vi "Write file.vi"() -> ()   [LabVIEW 2019]
panel:
  out "text":string
  in  "stop":bool
  in  "Enable 3":bool=TRUE caption="Enable"
  out "AZ1 Actual Current (A)":dbl format="%.2f"
  out "AZ2 EN ST":bool=TRUE
  out "AZ Axis POS (Arecsec)":dbl
  out "AZ1 EN ST":bool=TRUE
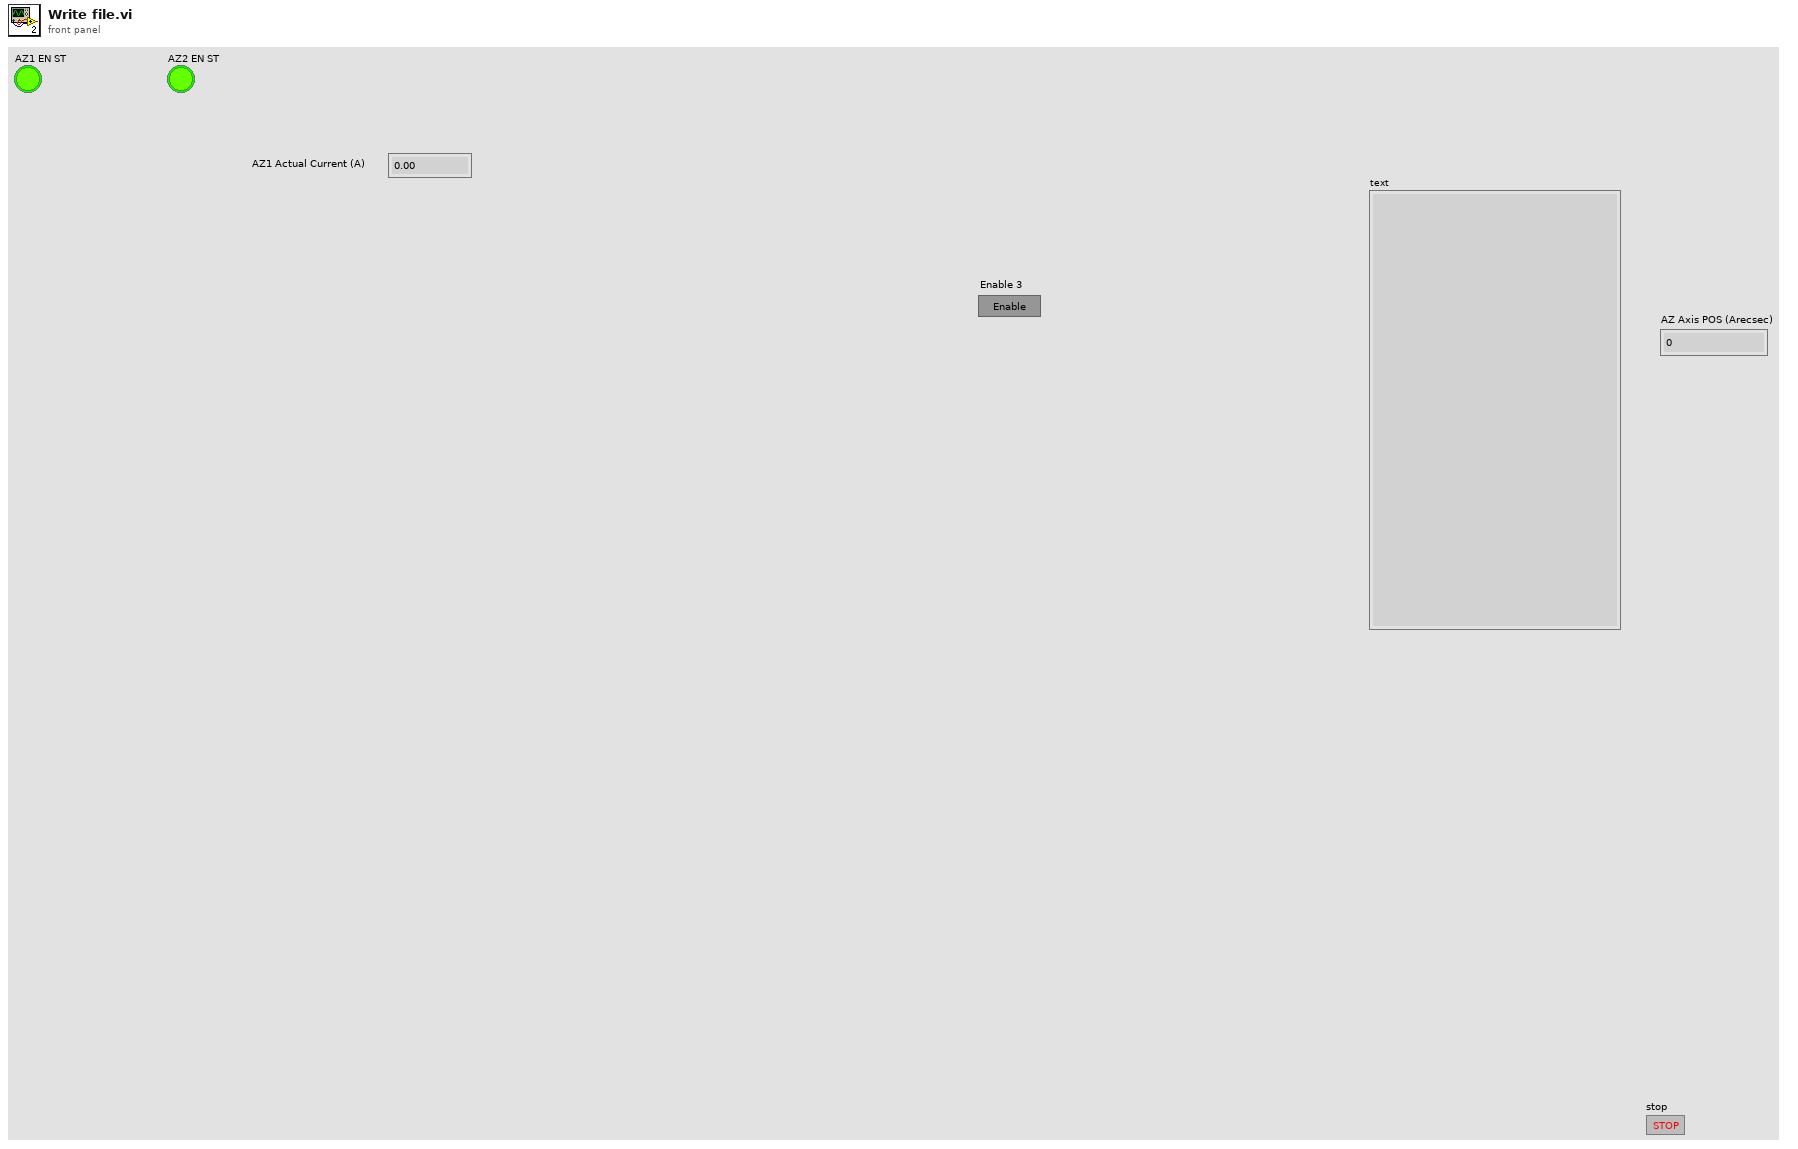
[diagram p1: front panel]
types:
  T1 = enum16{"open", "replace", "create", "open or create", "replace or create", "replace or create with confirmation"}
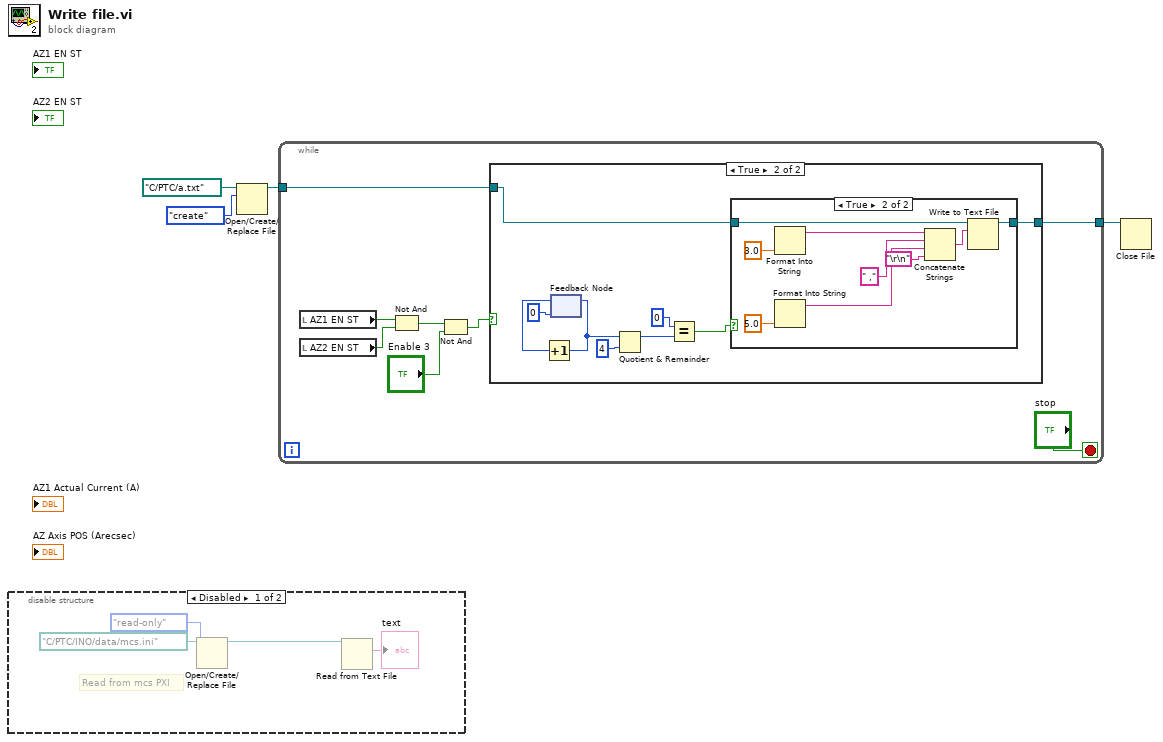
[diagram p0: block diagram]
diagram:
  n1 = disable-structure shown="Disabled" {
    frame Disabled {
      # "Read from mcs PXI"
      n2 = Open/Create/Replace File(file path (use dialog)=path "C:/PTC/INO/data/mcs.ini", access (0:read/write)=enum16{"read/write", "read-only", "write-only"}."read-only") -> (refnum out=w7:refnum<file>)  [unwired: 4 in, 2 out]
      n3 = Read from Text File(file (use dialog)=w7) -> (text=→"text":string)  [unwired: 3 in, 3 out]
    }
    frame Enabled {
    }
  }
  n4 = Open/Create/Replace File(file path (use dialog)=path "C:/PTC/a.txt" ("file path (dialog if empty)"), operation (0:open)=T1."create") -> (refnum out=w4:refnum<file>)  [unwired: 4 in, 2 out]
  n5 = while {
    tunnel: w4 -> [w10]
    tunnel: [w9] -> w1
    stop <- "stop" stop-if-true
    n6 = local read "AZ1 EN ST"() -> (w16:bool)
    n7 = local read "AZ2 EN ST"() -> (w15:bool)
    n8 = Not And(1:w15, 2:w16) -> (0:w14:bool)
    n9 = Not And(1:"Enable 3", 2:w14) -> (0:w12:bool)
    n10 = case shown="True" w12 {
      tunnel: w10 -> [_ w18]
      tunnel: [_ w17] -> w9
      frame False {
      }
      frame True {
        n11 = feedback #1(0) -> (w24:i32)
        n12 = Increment(x=w24) -> (x+1=w22:i32)
        n13 = feedback-in #1(w22) -> ()
        n14 = Quotient & Remainder(x=w22, y=4) -> (x-y*floor(x/y)=w21:i32)  [unwired: 1 out]
        n15 = Equal?(x=0, y=w21) -> (x = y?=w19:bool)
        n16 = case shown="True" w19 {
          tunnel: w18 -> [_ w27]
          tunnel: [_ w26] -> w17
          frame False {
          }
          frame True {
            n17 = Format Into String(3.0) -> (resulting string=w32:string)  [unwired: 3 in, 1 out]
            n18 = Format Into String(5.0) -> (resulting string=w30:string)  [unwired: 3 in, 1 out]
            n19 = Concatenate Strings(w32, " ," ("string"), w30, "\r\n") -> (w28:string)
            n20 = Write to Text File(file (use dialog)=w27, text=w28) -> (refnum out=w26:refnum<file>)  [unwired: 2 in, 2 out]
          }
        }
      }
    }
  }
  n21 = Close File(refnum=w1) -> ()  [unwired: 1 in, 2 out]
